vi "PrgGet.vi"(7 "error in (no error)":errorcluster, 10 "Program in":refnum<class "Program.lvclass">) -> (0 "error out":errorcluster, 1 "Tag":string, 2 "An Array of SEQ":refnum<class "Sequence.lvclass">[](array[class]), 3 "Program out":refnum<class "Program.lvclass">)   [LabVIEW 2012, in "Program.lvclass"]
uses:
  Program.lvclass
  Sequence.lvclass
  Program.lvclass/Program.ctl
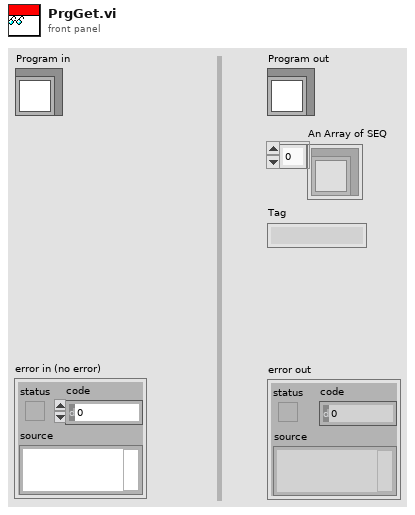
[diagram p1: front panel]
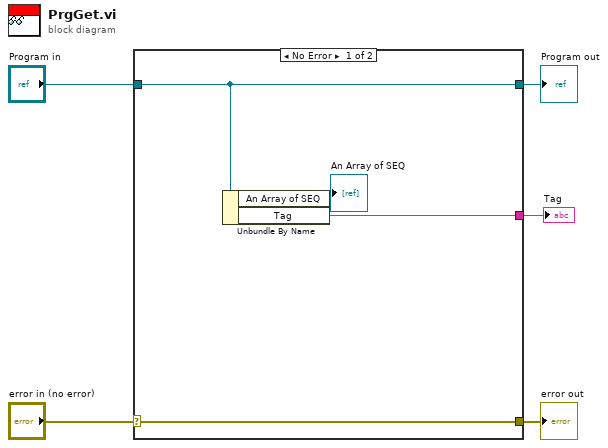
[diagram p0: block diagram]
diagram:
  n1 = case shown="No Error" "error in (no error)" {
    selector: "error in (no error)" -> [w8 w9]
    tunnel: [w8 w9] -> w4
    tunnel: [w7 w10] -> w2
    tunnel: "Program in" -> [w7 w10]
    tunnel: [w6 _] -> w1
    frame No Error {
      n2 = Unbundle By Name(w7) -> ("Tag"=w6:string)  [unwired: 1 out]
    }
    frame Error {
    }
  }
  "error out" <- w4
  "Program out" <- w2
  "Tag" <- w1
